vi "String Parser.vi"(8 "Error in (no error)":errorcluster, 10 "File Type":string, 11 "raw string":string) -> (0 "Error out":errorcluster, 3 "Array":T1(array[cluster]))   [LabVIEW 2017, in "Text based Communications Test.lvlib" / "Text based Communications Test.lvclass"]
uses:
  Text based Communications Test.lvclass
  <vilib>/regexp/Match Regular Expression.xnode
panel:
  # "This parser support both of the given file formats\n(*.txt & *.json)"
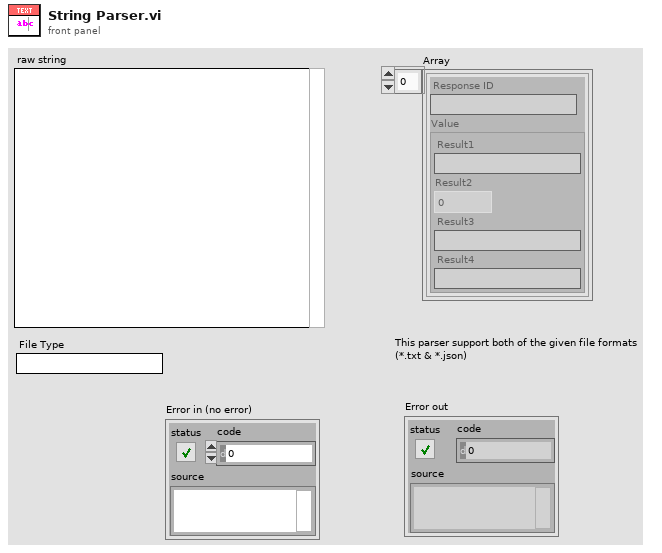
[diagram p1: front panel]
types:
  T1 = cluster{"Response ID":string, "Value":cluster{"Result1":string, "Result2":dbl, "Result3":string, "Result4":string}}[]
  T2 = cluster{"Response ID":string, "Value":cluster{"Result1":string, "Result2":dbl, "Result3":string, "Result4":string}}
  T3 = cluster{"Result1":string, "Result2":dbl, "Result3":string, "Result4":string}
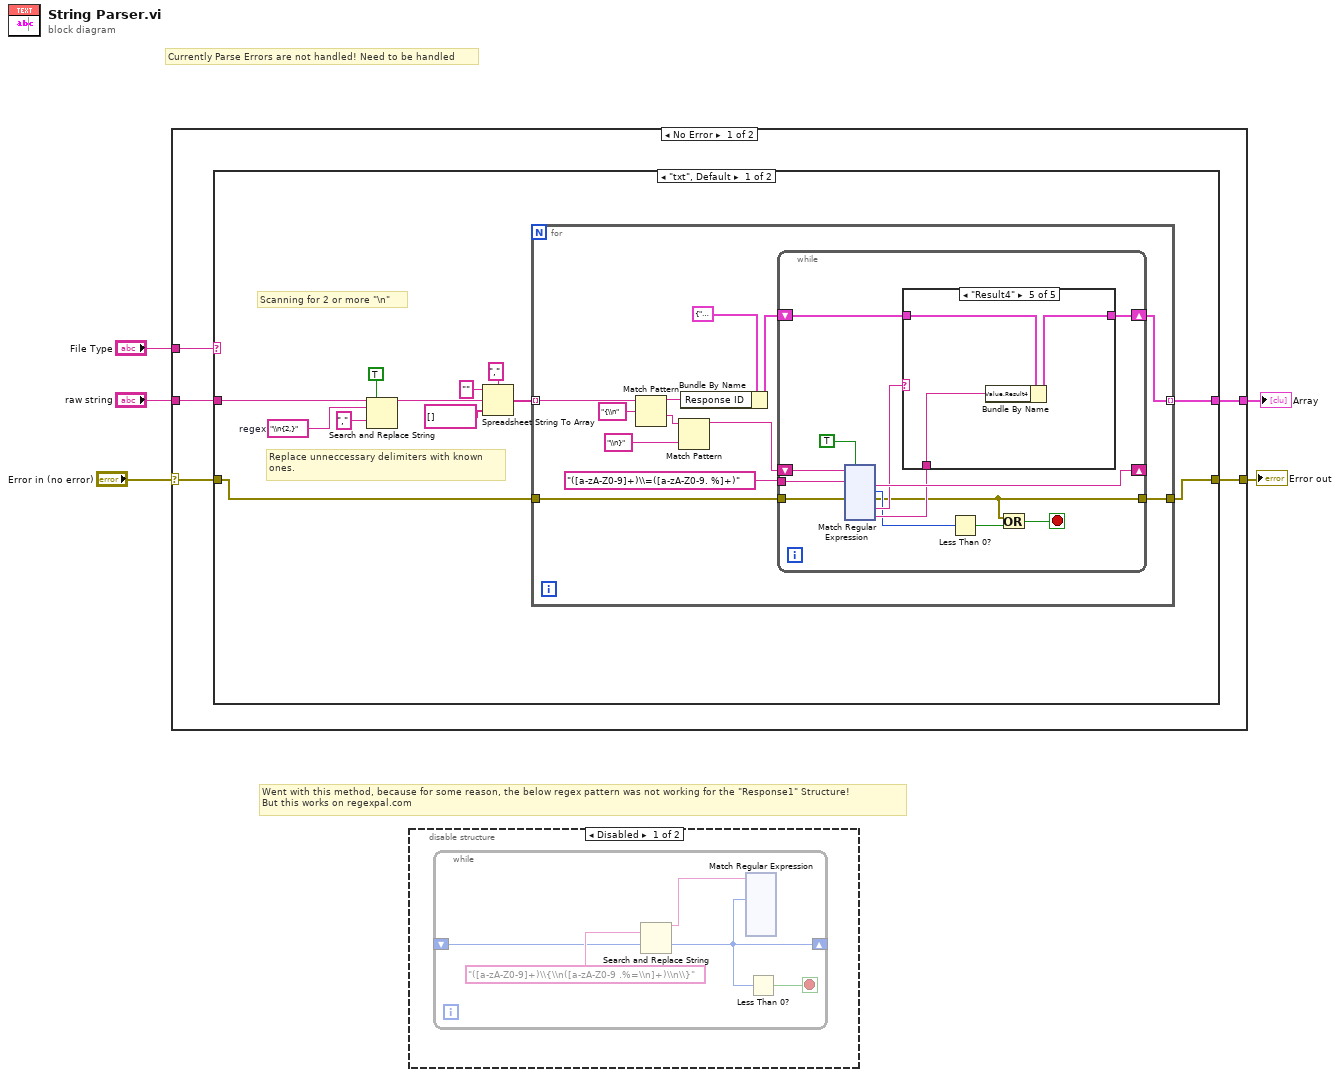
[diagram p0: block diagram]
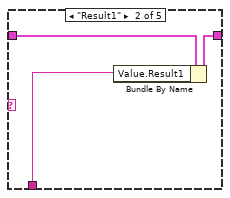
[diagram p4: hidden frame]
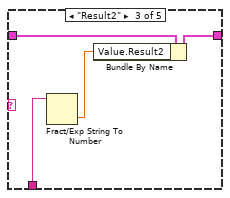
[diagram p5: hidden frame]
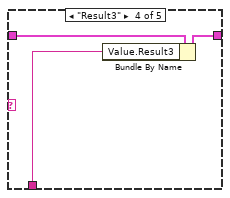
[diagram p6: hidden frame]
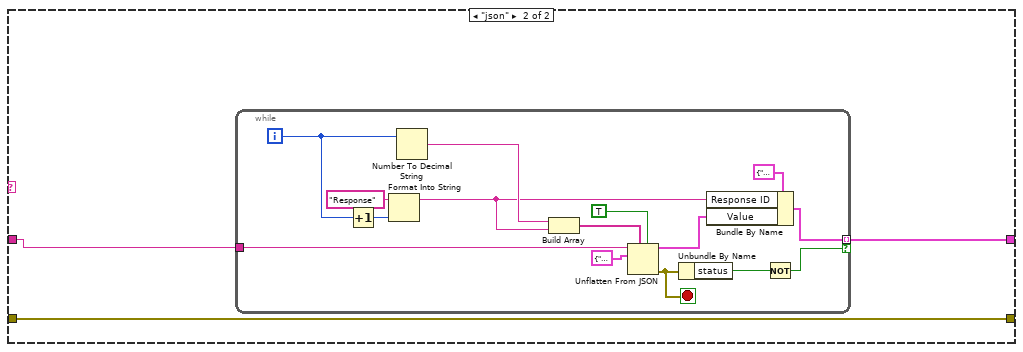
[diagram p7: hidden frame]
diagram:
  # "Went with this method, because for some reason, the below regex pattern was not working for the \"Response1\" Structure! \nBut this works on regexpal.com"
  # "Currently Parse Errors are not handled! Need to be handled"
  n1 = case shown="No Error" "Error in (no error)" {
    selector: "Error in (no error)" -> [w7 w197]
    tunnel: [w10 _] -> w5
    tunnel: "File Type" -> [w9 _]
    tunnel: "raw string" -> [w8 _]
    tunnel: [w6 w197] -> w1
    frame No Error {
      n2 = case shown="\"txt\", Default" w9 {
        tunnel: w8 -> [w22 w181]
        tunnel: [w13 w180] -> w10
        tunnel: w7 -> [w12 w179]
        tunnel: [w11 w179] -> w6
        frame "txt", Default {
          w21 = "\\n{2,}"  # regex
          # "Scanning for 2 or more \"\\n\""
          # "Replace unneccessary delimiters with known\nones."
          n3 = Search and Replace String(replace all?=TRUE ("replace all? (F)"), input string=w22, search string=w21, replace string="," ("replace string (\"\")")) -> (result string=w15:string)  [unwired: 4 in, 3 out]
          n4 = Spreadsheet String To Array(delimiter (Tab)=",", format string="", spreadsheet string=w15, array type (2D Dbl)=string[] [] ("spreadsheet string")) -> (array=w14:string[])
          n5 = for {
            tunnel: w14 -> [w34] mode=indexing
            tunnel: [w25] -> w13 mode=indexing
            tunnel: w12 -> [w24]
            tunnel: [w23] -> w11
            n6 = Match Pattern(string=w34, regular expression="{\\n") -> (before substring=w32:string, after substring=w31:string)  [unwired: 1 in, 2 out]
            n7 = Match Pattern(string=w31, regular expression="\\n}") -> (before substring=w26:string)  [unwired: 1 in, 3 out]
            n8 = Bundle By Name(cluster=T2 {"Response ID"="", "Value"={"Result1"="", "Result2"=0.0, "Result3"="", "Result4"=""}}, "Response ID"=w32) -> (w28:T2)
            n9 = while {
              tunnel: "([a-zA-Z0-9]+)\\=([a-zA-Z0-9. %]+)" ("regular expression") -> [w46]
              shift-right: [w42] -> _
              shift-left: w26 -> [w45]
              shift-right: [w43] -> w25
              shift-left: w28 -> [w44]
              tunnel: w24 -> [w38]
              tunnel: [w37] -> w23
              stop <- w35 stop-if-true
              n10 = xnode "Match Regular Expression"("input string"=w45, "regular expression"=w46, "error in"=w38, "ignore case? (F)"=TRUE) -> ("after match"=w42:string, "offset past match"=w39:i32, "error out"=w37:errorcluster, "submatch 1"=w41:string, "submatch 2"=w40:string)  [unwired: 2 in, 2 out]
              n11 = case shown="\"Result4\"" w41 {
                tunnel: w44 -> [w48 w51 w55 w58 w61]
                tunnel: [w48 w50 w54 w57 w60] -> w43
                tunnel: w40 -> [_ w49 w53 w56 w59]
                frame "False", Default {
                }
                frame "Result1" {
                  n12 = Bundle By Name(cluster=w51, "Value.Result1"=w49) -> (w50:T2)
                }
                frame "Result2" {
                  n13 = Fract/Exp String To Number(string=w53) -> (number=w52:dbl)  [unwired: 3 in, 1 out]
                  n14 = Bundle By Name(cluster=w55, "Value.Result2"=w52) -> (w54:T2)
                }
                frame "Result3" {
                  n15 = Bundle By Name(cluster=w58, "Value.Result3"=w56) -> (w57:T2)
                }
                frame "Result4" {
                  n16 = Bundle By Name(cluster=w61, "Value.Result4"=w59) -> (w60:T2)
                }
              }
              n17 = Less Than 0?(x=w39) -> (x < 0?=w36:bool)
              n18 = Or(x=w37, y=w36) -> (x .or. y?=w35:bool)
            }
          }
        }
        frame "json" {
          n19 = while {
            tunnel: w181 -> [w196]
            tunnel: [w189] -> w180 mode=indexing if=w191
            i -> [w187]
            stop <- w193 stop-if-true
            n20 = Increment(x=w187) -> (x+1=w183:i32)
            n21 = Format Into String(initial string="Response", w183) -> (resulting string=w184:string)  [unwired: 2 in, 1 out]
            n22 = Number To Decimal String(number=w187) -> (decimal integer string=w186:string)  [unwired: 1 in]
            n23 = Build Array(w186, w184) -> (w185:string[])
            n24 = Unflatten From JSON(path=w185, enable LabVIEW extensions? (T)=TRUE, JSON string=w196, type and defaults=T3 {"Result1"="", "Result2"=0.0, "Result3"="", "Result4"=""}) -> (value=w188:T3, error out=w193:errorcluster)  [unwired: 3 in]
            n25 = Unbundle By Name(w193) -> ("status"=w192:bool)
            n26 = Bundle By Name(cluster=T2 {"Response ID"="", "Value"={"Result1"="", "Result2"=0.0, "Result3"="", "Result4"=""}}, "Response ID"=w184, "Value"=w188) -> (w189:T2)
            n27 = Not(x=w192) -> (.not. x?=w191:bool)
          }
        }
      }
    }
    frame Error {
    }
  }
  "Array" <- w5
  "Error out" <- w1
  n28 = disable-structure shown="Disabled" {
    frame Disabled {
      n29 = while {
        shift-right: [w199] -> _
        shift-left: _ -> [w201]
        stop <- w198 stop-if-true
        n30 = Search and Replace String(search string="([a-zA-Z0-9]+)\\{\\n([a-zA-Z0-9 .%=\\n]+)\\n\\}", offset=w201) -> (result string=w200:string, offset past replacement=w199:i32)  [unwired: 6 in, 2 out]
        n31 = xnode "Match Regular Expression"("input string"=w200, "offset (0)"=w199) -> ()  [unwired: 4 in, 8 out]
        n32 = Less Than 0?(x=w199) -> (x < 0?=w198:bool)
      }
    }
    frame Enabled {
    }
  }
